vi "MALT get devices.vi"() -> ()   [LabVIEW 2018]
uses:
  <instrlib>/AltonTech MALT/AltonTech MALT200817.lvlib
panel:
  out "Devices":string[](array[string])
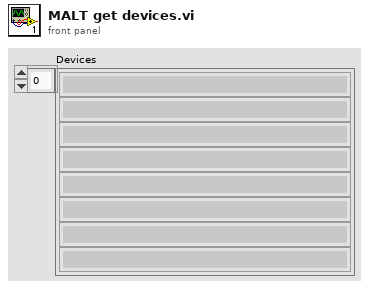
[diagram p1: front panel]
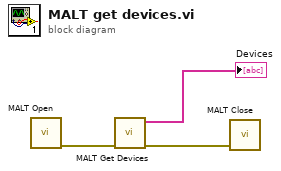
[diagram p0: block diagram]
diagram:
  n1 = call <instrlib>:"MALT Open.vi"() -> ("error out"=w2:errorcluster)  [unwired: 10 in, 1 out]
  n2 = call <instrlib>:"MALT Get Devices.vi"("error in"=w2) -> ("error out"=w1:errorcluster, "Devices"=→"Devices":string[])  [unwired: 9 in]
  n3 = call <instrlib>:"MALT Close.vi"("error in"=w1) -> ()  [unwired: 10 in, 1 out]
